vi "数组转换为字符串.vi"(10 "字符串数组":string[](array[string])) -> (2 "字符串":string)   [LabVIEW 2013]
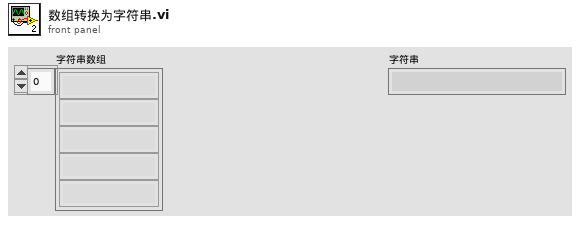
[diagram p1: front panel]
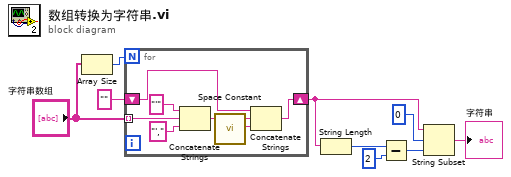
[diagram p0: block diagram]
diagram:
  n1 = Array Size(array="字符串数组") -> (size(s)=w9:i32)
  n2 = for {
    N: w9 -> [_]
    tunnel: "字符串数组" -> [w16] mode=indexing
    shift-right: [w11] -> w6
    shift-left: "" -> [w13]
    n3 = Concatenate Strings("'" ("字符串"), w16, "'," ("字符串")) -> (w12:string)
    n4 = call <vilib>:"Space Constant.vi"() -> ("String"=w10:string)
    n5 = Concatenate Strings(w13, w12, w10) -> (w11:string)
  }
  n6 = String Length(string=w6) -> (length=w4:i32)
  n7 = Subtract(x=w4, y=2) -> (x-y=w2:i32)
  n8 = String Subset(string=w6, offset (0)=0 ("偏移量(0)"), length (rest)=w2) -> (substring=→"字符串":string)
